vi "Actor Core.vi"(8 "error in":errorcluster, 11 "Nested in":refnum<class "MQTT_Client_Actor.lvclass">) -> (0 "error out":errorcluster, 3 "Actor out":refnum<class "Actor.lvclass">)   [LabVIEW 2018, in "MQTT_Client_Actor.lvlib" / "MQTT_Client_Actor.lvclass"]
doc: "(<B>Filename</B>: Actor Framework.lvlib:Actor.lvclass:Actor Core.vi)\n\nReceives messages to the actor, reacts to them, and initiates any error handling that may shut the actor down.\n\nDescendant classes may override this VI to append parallel tasks for the actor to complete while it handles messages. Overrides use the Call Parent Method node."
uses:
  MQTT_Client_Actor.lvclass
  D:/Program Files (x86)/National Instruments/LabVIEW 2018/vi.lib/ActorFramework/Actor/Actor.lvclass
  <vilib>/ActorFramework/Actor/Actor.lvclass
  CreateClient.ctl
  <vilib>/LabVIEW Open Source Project/MQTT Control Packets/Control Packets/ControlPacket/QualityOfService -- enum.ctl
  <vilib>/LabVIEW Open Source Project/MQTT Client/Client class/Client.lvclass
  D:/Program Files (x86)/National Instruments/LabVIEW 2018/vi.lib/LabVIEW Open Source Project/MQTT Connection/MQTT_Base/Base Class/MQTT_Base.lvclass
  MQTT_Client_Actor.lvclass/MQTT_Client_Actor.ctl
  <vilib>/ActorFramework/Actor/Actor.lvclass/Actor.ctl
  <vilib>/ActorFramework/Message Enqueuer/Message Enqueuer.lvclass/Message Enqueuer.ctl
  <vilib>/LabVIEW Open Source Project/MQTT Client/Client class/Client.lvclass/Client.ctl
  <vilib>/LabVIEW Open Source Project/MQTT Connection/MQTT_Base/Base Class/MQTT_Base.lvclass/MQTT_Base.ctl
  <vilib>/LabVIEW Open Source Project/MQTT Control Packets/Control Packets/ControlPacket/ControlPacket.lvclass/ControlPacket.ctl
  <vilib>/LabVIEW Open Source Project/MQTT Control Packets/Control Packets/CONNECT/ConnectFlags -- cluster.ctl
  SubscribeClient.ctl
  PublishClient.ctl
  <vilib>/ActorFramework/Message Enqueuer/Init from Existing Queue.vi
  <vilib>/ActorFramework/Message Enqueuer/Enqueue.vi
  <vilib>/ActorFramework/Stop Msg/Stop Msg.lvclass
  D:/Program Files (x86)/National Instruments/LabVIEW 2018/vi.lib/ActorFramework/Message/Message.lvclass
  <vilib>/LabVIEW Open Source Project/MQTT Control Packets/Control Packets/PUBLISH/PUBLISH.lvclass
  D:/Program Files (x86)/National Instruments/LabVIEW 2018/vi.lib/LabVIEW Open Source Project/MQTT Control Packets/Control Packets/ControlPacket/ControlPacket.lvclass
  <vilib>/LabVIEW Open Source Project/Connection/Connection.TCP/Connection.TCP.lvclass
  D:/Program Files (x86)/National Instruments/LabVIEW 2018/vi.lib/LabVIEW Open Source Project/Connection/Connection/Connection.lvclass
  <vilib>/ActorFramework/Message Priority Queue/Priority Enqueue.vi
  <vilib>/ActorFramework/Message Enqueuer/Message Enqueuer.lvclass
  <vilib>/LabVIEW Open Source Project/MQTT Connection/MQTT_Base/Base Class/MQTT_Base.lvclass
  <vilib>/LabVIEW Open Source Project/MQTT Control Packets/Control Packets/ControlPacket/ControlPacket.lvclass
  MQTT_Client_Actor Messages/1_CreateClient Msg/1_CreateClient Msg.lvclass
  <vilib>/LabVIEW Open Source Project/MQTT Control Packets/Control Packets/CONNECT/CONNECT.lvclass
  MQTT_Client_Actor Messages/2_Subscribe Msg/2_Subscribe Msg.lvclass
  MQTT_Client_Actor Messages/3_UpdateSubscribeList Msg/3_UpdateSubscribeList Msg.lvclass
  MQTT_Client_Actor Messages/4_Publish Msg/4_Publish Msg.lvclass
panel:
  in  "RETAIN":bool
  out "SubscribeLists":i32(listbox)
  in  "Topic Name":string="Topic"
  in  "QoS":T1=enum."1 (At Least Once)"
  in  "Create":T2={"address"="localhost", "port"=1883, "UserName"="", "Pwd"=""}
  out "ServerStatus":bool
  in  "CreateClient":bool
  in  "UnSubscribe":bool
  out "ReceivedData":i32(listbox)
  in  "Subscribe":bool
  in  "Publish":bool
  out "Published":bool
  in  "Data":string="12345"
  in  "DisConnect":bool
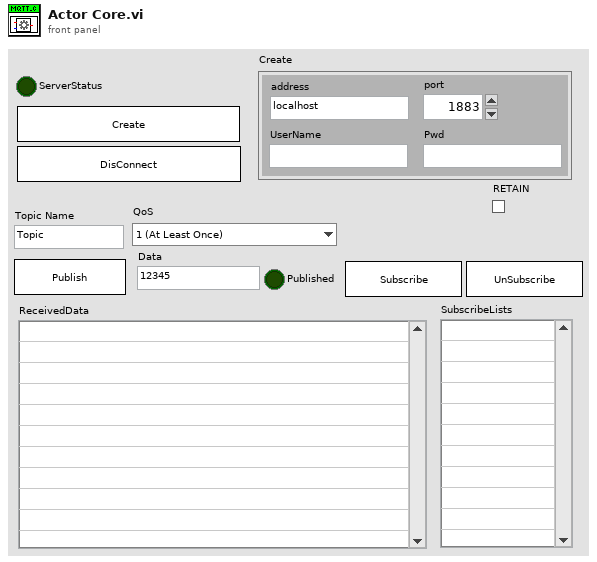
[diagram p1: front panel]
types:
  T1 = typedef "MQTT_Control_Packets.lvlib/ControlPacket.lvclass/QualityOfService -- enum.ctl" = enum16{"0 (At Most Once)", "1 (At Least Once)", "2 (Exactly Once)"}
  T2 = typedef "MQTT_Client_Actor.lvlib/MQTT_Client_Actor.lvclass/CreateClient.ctl" = cluster{"address":string, "port":u16, "UserName":string, "Pwd":string}
  T3 = typedef "MQTT Client.lvlib/Client.lvclass/Public Events -- cluster.ctl" = cluster{"Connection Status":refnum<user-event>, "Connected":refnum<user-event>, "Application Message":refnum<user-event>}
  T4 = cluster{"Stop":refnum<user-event>, "Create":refnum<user-event>, "Subscribe":refnum<user-event>, "Init":refnum<user-event>, "Publish":refnum<user-event>}
  T5 = typedef "MQTT Base.lvlib/MQTT_Base.lvclass/Public Events -- cluster.ctl" = cluster{"Stop Event":refnum<user-event>, "Error Event":refnum<user-event>, "Inbound Message":refnum<user-event>}
  T6 = typedef "MQTT_Control_Packets.lvlib/CONNECT.lvclass/ConnectFlags -- cluster.ctl" = cluster{"Reserved":bool, "Clean Session":bool, "Will Flag":bool, "Will QoS 1":bool, "Will QoS 2":bool, "Will Retain":bool, "Password Flag":bool, "User Name Flag":bool}
  T7 = cluster{"Will Topic":string, "Will Message":string, "Username":string, "Password":string}
  T8 = typedef "MQTT_Client_Actor.lvlib/MQTT_Client_Actor.lvclass/SubscribeClient.ctl" = cluster{"Topic Name":string, "QoS":T1, "T:Subscribe":bool}
  T9 = typedef "MQTT_Client_Actor.lvlib/MQTT_Client_Actor.lvclass/PublishClient.ctl" = cluster{"Topic Name":string, "QoS":T1, "RETAIN":bool, "Topic Data":string}
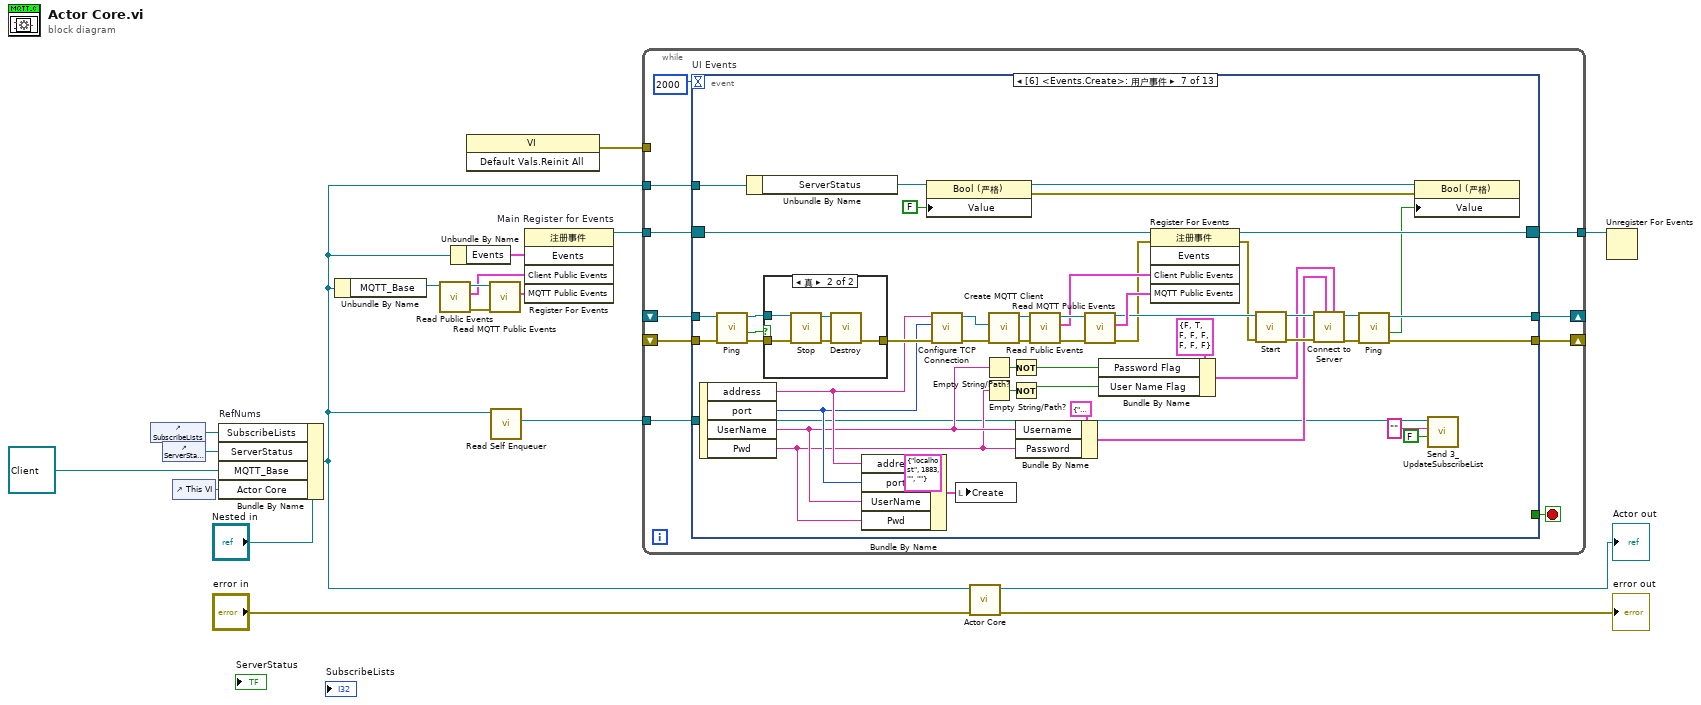
[diagram p0: block diagram]
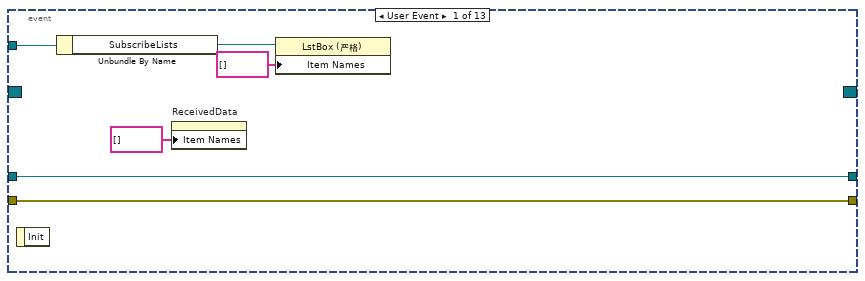
[diagram p2: hidden frame]
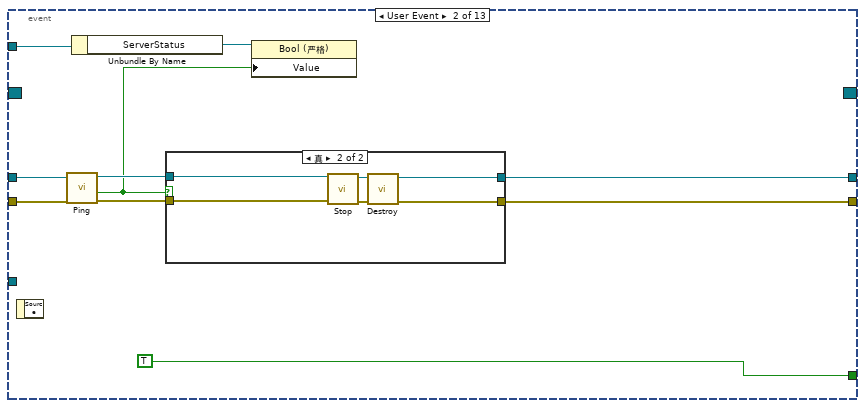
[diagram p3: hidden frame]
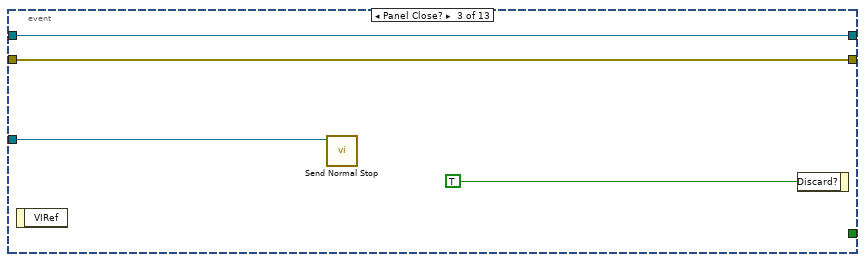
[diagram p5: hidden frame]
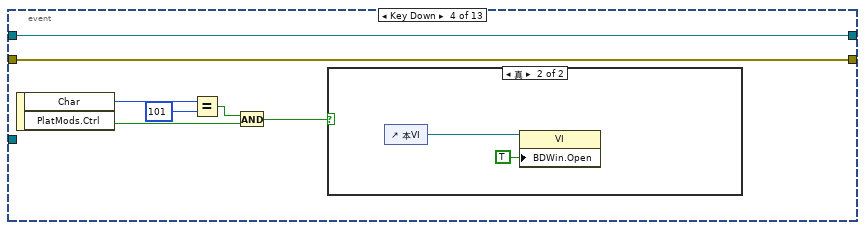
[diagram p6: hidden frame]
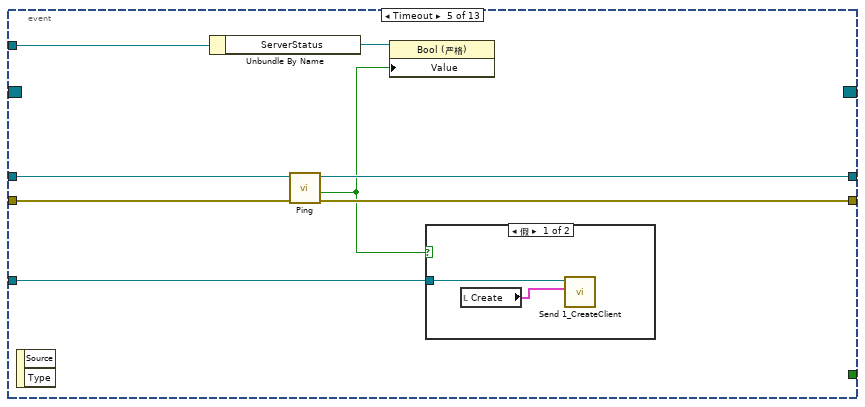
[diagram p8: hidden frame]
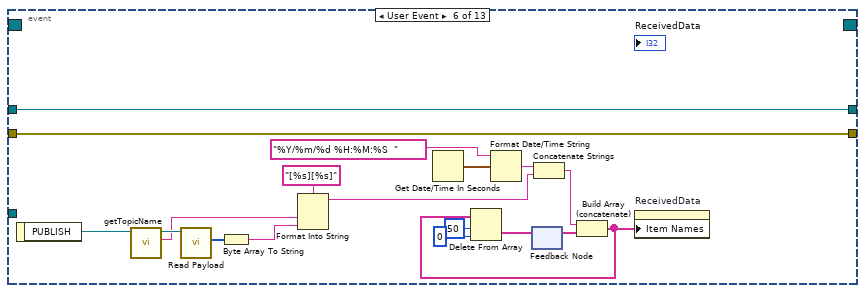
[diagram p10: hidden frame]
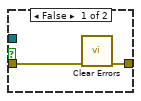
[diagram p11: hidden frame]
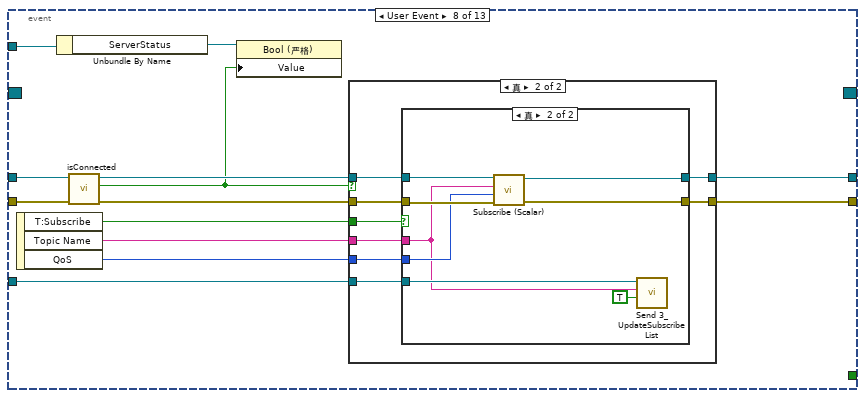
[diagram p12: hidden frame]
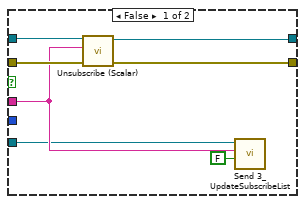
[diagram p14: hidden frame]
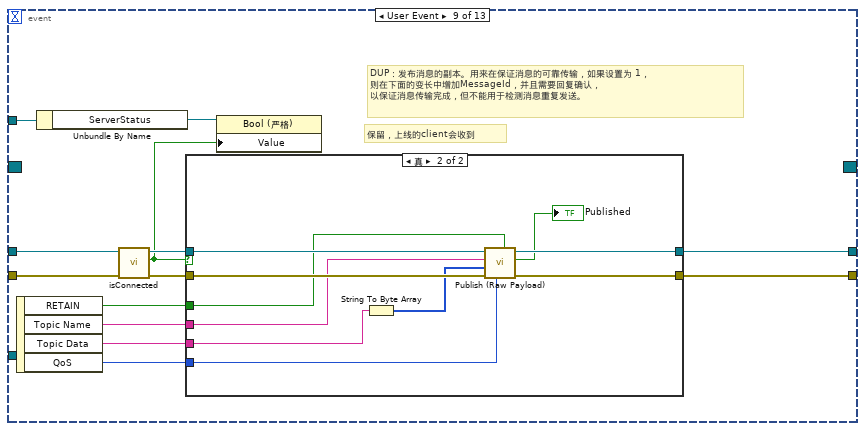
[diagram p15: hidden frame]
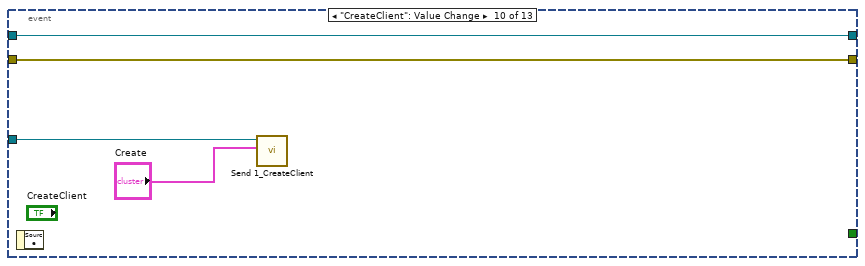
[diagram p17: hidden frame]
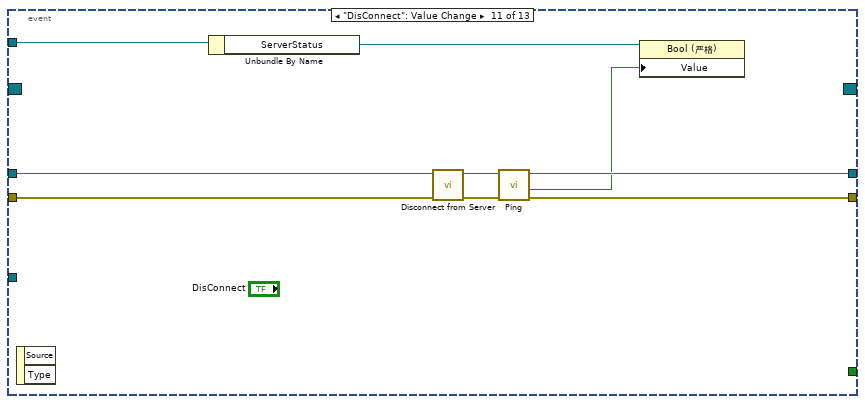
[diagram p18: hidden frame]
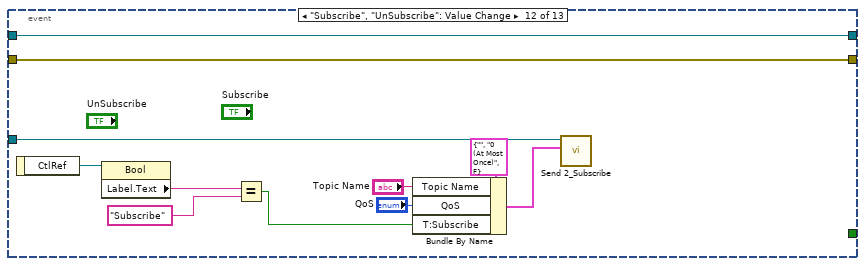
[diagram p19: hidden frame]
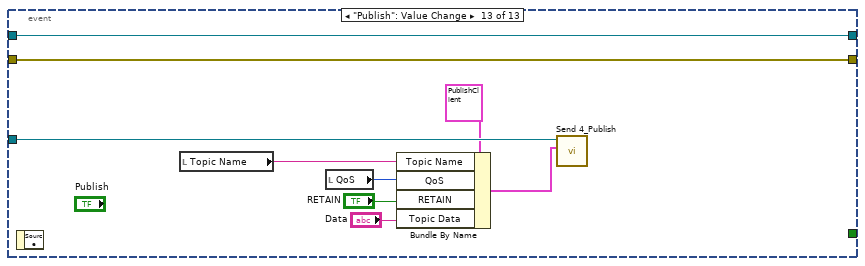
[diagram p20: hidden frame]
diagram:
  n1 = control-ref of="SubscribeLists"() -> (w2:refnum<vi>)
  n2 = control-ref of="ServerStatus"() -> (w4:refnum<vi>)
  n3 = control-ref of="This VI"() -> (w12:refnum<vi>)
  n4 = Bundle By Name "RefNums"(cluster="Nested in", "SubscribeLists"=w2, "ServerStatus"=w4, "MQTT_Base"=refnum<class "Client.lvclass"> refnum, "Actor Core"=w12) -> (w3:refnum<class "MQTT_Client_Actor.lvclass">)
  n5 = Unbundle By Name(w3) -> ("MQTT_Base"=w7:refnum<class "Client.lvclass">)
  n6 = call <vilib>:"Read Public Events.vi"("Client in"=w7) -> ("error out"=w8:errorcluster, "Client Public Events"=w6:T3, "Client out"=w9:refnum<class "Client.lvclass">)  [unwired: 8 in]
  n7 = Unbundle By Name(w3) -> ("Events"=w16:T4)
  n8 = invoke class="VI" method="Default Vals.Reinit All"() -> (error out=w1:errorcluster)  [unwired: 3 in, 2 out]
  n9 = call <vilib>:"Read MQTT Public Events.vi"("error in (no error)"=w8, "MQTT_Base in"=w9) -> ("MQTT Public Events"=w5:T5)  [unwired: 7 in, 2 out]
  n10 = call <vilib>:"Read Self Enqueuer.vi"("Actor"=w3) -> ("Self Enqueuer"=w14:refnum<class "Message Enqueuer.lvclass">)  [unwired: 10 in]
  n11 = register-events "Main Register for Events"(w16, w6, w5) -> (reference out=w17:refnum<event-registration>)  [unwired: 2 in, 1 out]
  n12 = while {
    tunnel: w17 -> [w29]
    tunnel: [w27] -> w15
    tunnel: w14 -> [w26]
    shift-right: [w25] -> _
    shift-left: _ -> [w21]
    shift-right: [w24] -> _
    shift-left: _ -> [w22]
    tunnel: w3 -> [w20]
    tunnel: w1 -> [_]
    stop <- w28 stop-if-true
    n13 = event "UI Events" shown="[6] <Events.Create>: 用户事件" {
      selector: w29 -> [_ _ _ _ _ _ w137 _ _ _ _ _ _]
      dyn-events: [_ _ _ _ _ _ w134 _ _ _ _ _ _] -> w27
      timeout: 2000 -> [_ _ _ _ _ _ _ _ _ _ _ _ _]
      tunnel: [_ TRUE _ _ _ _ _ _ _ _ _ _ _] -> w28
      tunnel: w26 -> [_ _ w56 _ w68 _ w95 w150 _ w213 _ w234 w243]
      tunnel: [w35 w40 w54 w64 w72 w91 w110 w157 w195 w216 w220 w236 w245] -> w25
      tunnel: [w34 w39 w55 w63 w71 w90 w125 w158 w196 w215 w221 w235 w244] -> w24
      tunnel: w22 -> [w34 w44 w55 w63 w74 w90 w123 w160 w198 w215 w225 w235 w244]
      tunnel: w21 -> [w35 w43 w54 w64 w73 w91 w122 w159 w197 w216 w224 w236 w245]
      tunnel: w20 -> [w32 w37 _ _ w69 _ w116 w155 w193 _ w218 _ _]
      event User Event {
        n14 = event-data() -> ()  [unwired: 1 in, 1 out]
        n15 = Unbundle By Name(w32) -> ("SubscribeLists"=w31:refnum<vi>)
        n16 = property on="ReceivedData" class="LstBox (严格)"("Item Names"=string[] [] ("项名")) -> ()  [unwired: 2 in, 2 out]
        n17 = property class="LstBox (严格)"(reference=w31, "Item Names"=string[] [] ("项名")) -> ()  [unwired: 1 in, 2 out]
      }
      event User Event {
        n18 = event-data() -> ()  [unwired: 1 in, 1 out]
        n19 = call <vilib>:"Ping.vi"("error in (no error)"=w43, "Client in"=w44) -> ("error out"=w41:errorcluster, "Server responded"=w36:bool, "Client out"=w42:refnum<class "Client.lvclass">)  [unwired: 6 in, 1 out]
        n20 = Unbundle By Name(w37) -> ("ServerStatus"=w38:refnum<vi>)
        n21 = case shown="真" w36 {
          tunnel: w42 -> [w47 w51]
          tunnel: w41 -> [w46 w50]
          tunnel: [w46 w49] -> w40
          tunnel: [w47 w48] -> w39
          frame False {
          }
          frame True {
            n22 = call <vilib>:"Stop.vi"("error in (no error)"=w50, "MQTT_Base in"=w51) -> ("error out"=w52:errorcluster, "MQTT_Base out"=w53:refnum<class "Client.lvclass">)  [unwired: 7 in, 1 out]
            n23 = call <vilib>:"Destroy.vi"("error in (no error)"=w52, "MQTT_Base in"=w53) -> ("error out"=w49:errorcluster, "MQTT_Base out"=w48:refnum<class "Client.lvclass">)  [unwired: 8 in]
          }
        }
        n24 = property class="Bool (严格)"(reference=w38, "Value"=w36) -> ()  [unwired: 1 in, 2 out]
      }
      event Panel Close? {
        n25 = event-data() -> ()  [unwired: 1 in, 1 out]
        n26 = call <vilib>:"Send Normal Stop.vi"("Message Enqueuer"=w56) -> ()  [unwired: 10 in, 1 out]
        n27 = event-data("Discard?"=TRUE) -> ()  [unwired: 1 in, 1 out]
      }
      event Key Down {
        n28 = event-data() -> ("Char"=w59:i16, "PlatMods.Ctrl"=w58:bool)  [unwired: 1 in]
        n29 = Equal?(x=w59, y=i16 101) -> (x = y?=w61:bool)
        n30 = And(x=w61, y=w58) -> (x .and. y?=w60:bool)
        n31 = case shown="真" w60 {
          frame False {
          }
          frame True {
            n32 = control-ref of="本VI"() -> (w66:refnum<vi>)
            n33 = property class="VI"(reference=w66, "BDWin.Open"=TRUE ("程序框图窗口:打开")) -> ()  [unwired: 1 in, 2 out]
          }
        }
      }
      event Timeout {
        n34 = event-data() -> ()  [unwired: 1 in, 2 out]
        n35 = Unbundle By Name(w69) -> ("ServerStatus"=w70:refnum<vi>)
        n36 = call <vilib>:"Ping.vi"("error in (no error)"=w73, "Client in"=w74) -> ("error out"=w72:errorcluster, "Server responded"=w67:bool, "Client out"=w71:refnum<class "Client.lvclass">)  [unwired: 6 in, 1 out]
        n37 = property class="Bool (严格)"(reference=w70, "Value"=w67) -> ()  [unwired: 1 in, 2 out]
        n38 = case shown="假" w67 {
          tunnel: w68 -> [w76 _]
          frame False {
            n39 = local read "Create"() -> (w75:T2)
            n40 = call "Send 1_CreateClient.vi"("Create"=w75, "Message Enqueuer in"=w76) -> ()  [unwired: 8 in, 2 out]
          }
          frame True {
          }
        }
      }
      event User Event {
        n41 = event-data() -> ("PUBLISH"=w92:refnum<class "PUBLISH.lvclass">)  [unwired: 1 in]
        n42 = call <vilib>:"getTopicName.vi"("PUBLISH in"=w92) -> ("Topic"=w80:string, "PUBLISH out"=w93:refnum<class "PUBLISH.lvclass">)  [unwired: 8 in, 1 out]
        n43 = call <vilib>:"Read Payload.vi"("ControlPacket in"=w93) -> ("Payload"=w94:u8[])  [unwired: 9 in, 1 out]
        n44 = Byte Array To String(unsigned byte array=w94) -> (string=w79:string)
        n45 = Format Into String(format string="[%s][%s]" ("格式字符串"), w80, w79) -> (resulting string=w77:string)  [unwired: 2 in, 1 out]
        n46 = Get Date/Time In Seconds() -> (seconds since 1Jan1904=w89:timestamp)
        n47 = Format Date/Time String(time format string (%c)="%Y/%m/%d %H:%M:%S  " ("时间格式字符串(%c)"), seconds (now)=w89) -> (date/time string=w88:string)  [unwired: 1 in]
        n48 = feedback #1() -> (w85:string[])  [unwired: 1 in]
        n49 = Concatenate Strings(w88, w77) -> (w86:string)
        n50 = Build Array (concatenate)(w86, w85) -> (w81:string[])
        n51 = Delete From Array(array=w81, length=50 ("长度"), index=0 ("索引")) -> (deleted portion=w82:string[])  [unwired: 1 out]
        n52 = feedback-in #1(w82) -> ()
        n53 = property on="ReceivedData" class="LstBox (严格)"("Item Names"=w81) -> ()  [unwired: 2 in, 2 out]
      }
      event User Event {
        n54 = event-data() -> ("address"=w101:string, "port"=w100:u16, "UserName"=w99:string, "Pwd"=w98:string)  [unwired: 1 in]
        n55 = call <vilib>:"Ping.vi"("error in (no error)"=w122, "Client in"=w123) -> ("error out"=w119:errorcluster, "Server responded"=w121:bool, "Client out"=w120:refnum<class "Client.lvclass">)  [unwired: 6 in, 1 out]
        n56 = Unbundle By Name(w116) -> ("ServerStatus"=w114:refnum<vi>)
        n57 = case shown="真" w121 {
          tunnel: [w143 w147] -> w129
          tunnel: w120 -> [_ w146]
          tunnel: w119 -> [w144 w145]
          frame False {
            n58 = call <vilib>:"Clear Errors.vi"("error in (no error)"=w144) -> ("error out"=w143:errorcluster)  [unwired: 5 in, 1 out]
          }
          frame True {
            n59 = call <vilib>:"Stop.vi"("error in (no error)"=w145, "MQTT_Base in"=w146) -> ("error out"=w148:errorcluster, "MQTT_Base out"=w149:refnum<class "Client.lvclass">)  [unwired: 7 in, 1 out]
            n60 = call <vilib>:"Destroy.vi"("error in (no error)"=w148, "MQTT_Base in"=w149) -> ("error out"=w147:errorcluster)  [unwired: 8 in, 1 out]
          }
        }
        n61 = Bundle By Name(cluster=T2 {"address"="localhost", "port"=1883, "UserName"="", "Pwd"=""} ("Create"), "address"=w101, "port"=w100, "UserName"=w99, "Pwd"=w98) -> (w102:T2)
        n62 = property class="Bool (严格)"(reference=w114, "Value"=FALSE ("值")) -> (reference out=w113:refnum<vi>, error out=w112:errorcluster)  [unwired: 1 in]
        n63 = call <vilib>:"Configure TCP Connection.vi"("error in (no error)"=w129, "remote port (80)"=w100, "address (localhost)"=w101) -> ("error out"=w133:errorcluster, "Connection.TCP"=w138:refnum<class "Connection.TCP.lvclass">)  [unwired: 7 in]
        n64 = local write "Create"(w102) -> ()
        n65 = Empty String/Path?(string/path=w99) -> (empty?=w107:bool)
        n66 = Empty String/Path?(string/path=w98) -> (empty?=w106:bool)
        n67 = call <vilib>:"Create MQTT Client.vi"("error in (no error)"=w133, "Connection Configuration"=w138) -> ("error out"=w140:errorcluster, "Client out"=w142:refnum<class "Client.lvclass">)  [unwired: 8 in]
        n68 = Not(x=w107) -> (.not. x?=w105:bool)
        n69 = Not(x=w106) -> (.not. x?=w104:bool)
        n70 = Bundle By Name(cluster=T7 {"Will Topic"="", "Will Message"="", "Username"="", "Password"=""} ("Payload"), "Username"=w99, "Password"=w98) -> (w117:T7)
        n71 = call <vilib>:"Read Public Events.vi"("error in (no error)"=w140, "Client in"=w142) -> ("error out"=w139:errorcluster, "Client Public Events"=w136:T3, "Client out"=w141:refnum<class "Client.lvclass">)  [unwired: 7 in]
        n72 = call <vilib>:"Read MQTT Public Events.vi"("error in (no error)"=w139, "MQTT_Base in"=w141) -> ("error out"=w130:errorcluster, "MQTT Public Events"=w135:T5, "MQTT_Base out"=w132:refnum<class "Client.lvclass">)  [unwired: 7 in]
        n73 = Bundle By Name(cluster=T6 {"Reserved"=FALSE, "Clean Session"=TRUE, "Will Flag"=FALSE, "Will QoS 1"=FALSE, "Will QoS 2"=FALSE, "Will Retain"=FALSE, "Password Flag"=FALSE, "User Name Flag"=FALSE} ("Connect Flags"), "Password Flag"=w105, "User Name Flag"=w104) -> (w108:T6)
        n74 = register-events ("Main Register for Events")(reference=w137, error in=w130, w136, w135) -> (reference out=w134:refnum<event-registration>, error out=w131:errorcluster)  [unwired: 1 in]
        n75 = call <vilib>:"Start.vi"("error in (no error)"=w131, "MQTT_Base in"=w132) -> ("error out"=w127:errorcluster, "MQTT_Base out"=w128:refnum<class "Client.lvclass">)  [unwired: 7 in, 1 out]
        n76 = call <vilib>:"Connect to Server.vi"("Connect Flags"=w108, "Payload"=w117, "error in (no error)"=w127, "Client in"=w128) -> ("error out"=w124:errorcluster, "Client out"=w126:refnum<class "Client.lvclass">)  [unwired: 4 in, 2 out]
        n77 = call <vilib>:"Ping.vi"("error in (no error)"=w124, "Client in"=w126) -> ("error out"=w110:errorcluster, "Server responded"=w115:bool, "Client out"=w125:refnum<class "Client.lvclass">)  [unwired: 6 in, 1 out]
        n78 = property class="Bool (严格)"(reference=w113, error in=w112, "Value"=w115) -> ()  [unwired: 2 out]
        n79 = call "Send 3_UpdateSubscribeList.vi"("T:Add"=FALSE, "Topic"="", "Message Enqueuer in"=w95) -> ()  [unwired: 7 in, 2 out]
      }
      event User Event {
        n80 = event-data() -> ("T:Subscribe"=w153:bool, "Topic Name"=w152:string, "QoS"=w151:T1)  [unwired: 1 in]
        n81 = Unbundle By Name(w155) -> ("ServerStatus"=w156:refnum<vi>)
        n82 = call <vilib>:"isConnected.vi"("error in (no error)"=w159, "Client in"=w160) -> ("error out"=w161:errorcluster, "connected"=w154:bool, "Client out"=w162:refnum<class "Client.lvclass">)  [unwired: 7 in]
        n83 = property class="Bool (严格)"(reference=w156, "Value"=w154) -> ()  [unwired: 1 in, 2 out]
        n84 = case shown="真" w154 {
          tunnel: w162 -> [w164 w172]
          tunnel: w161 -> [w163 w171]
          tunnel: [w164 w170] -> w158
          tunnel: [w163 w169] -> w157
          tunnel: w153 -> [_ w168]
          tunnel: w152 -> [_ w167]
          tunnel: w151 -> [_ w166]
          tunnel: w150 -> [_ w165]
          frame False {
          }
          frame True {
            n85 = case shown="真" w168 {
              tunnel: [w177 w186] -> w170
              tunnel: [w176 w185] -> w169
              tunnel: w172 -> [w179 w187]
              tunnel: w171 -> [w178 w184]
              tunnel: w167 -> [w174 w180]
              tunnel: w166 -> [_ w183]
              tunnel: w165 -> [w173 w182]
              frame False {
                n86 = call <vilib>:"Unsubscribe (Scalar).vi"("error in (no error)"=w178, "Topic Filter"=w174, "Client in"=w179) -> ("error out"=w176:errorcluster, "Client out"=w177:refnum<class "Client.lvclass">)  [unwired: 6 in, 1 out]
                n87 = call "Send 3_UpdateSubscribeList.vi"("T:Add"=FALSE, "Topic"=w174, "Message Enqueuer in"=w173) -> ()  [unwired: 7 in, 2 out]
              }
              frame True {
                n88 = call <vilib>:"Subscribe (Scalar).vi"("error in (no error)"=w184, "QoS"=w183, "Topic Filter"=w180, "Client in"=w187) -> ("error out"=w185:errorcluster, "Client out"=w186:refnum<class "Client.lvclass">)  [unwired: 5 in, 1 out]
                n89 = call "Send 3_UpdateSubscribeList.vi"("T:Add"=TRUE, "Topic"=w180, "Message Enqueuer in"=w182) -> ()  [unwired: 7 in, 2 out]
              }
            }
          }
        }
      }
      event User Event {
        # "保留，上线的client会收到"
        # "DUP：发布消息的副本。用来在保证消息的可靠传输，如果设置为 1，\n则在下面的变长中增加MessageId，并且需要回复确认，\n以保证消息传输完成，但不能用于检测消息重复发送。"
        n90 = event-data() -> ("RETAIN"=w191:bool, "Topic Name"=w190:string, "Topic Data"=w189:string, "QoS"=w188:T1)  [unwired: 1 in]
        n91 = Unbundle By Name(w193) -> ("ServerStatus"=w194:refnum<vi>)
        n92 = call <vilib>:"isConnected.vi"("error in (no error)"=w197, "Client in"=w198) -> ("error out"=w200:errorcluster, "connected"=w192:bool, "Client out"=w199:refnum<class "Client.lvclass">)  [unwired: 7 in]
        n93 = case shown="真" w192 {
          tunnel: [w202 w211] -> w196
          tunnel: [w201 w210] -> w195
          tunnel: w199 -> [w202 w212]
          tunnel: w200 -> [w201 w209]
          tunnel: w191 -> [_ w206]
          tunnel: w190 -> [_ w205]
          tunnel: w189 -> [_ w204]
          tunnel: w188 -> [_ w203]
          frame False {
          }
          frame True {
            n94 = String To Byte Array(string=w204) -> (unsigned byte array=w208:u8[])
            n95 = call <vilib>:"Publish (Raw Payload).vi"("RETAIN"=w206, "QoS"=w203, "error in (no error)"=w209, "Binary Payload"=w208, "Topic Name"=w205, "Client in"=w212) -> ("error out"=w210:errorcluster, "Published"=→"Published":bool, "Client out"=w211:refnum<class "Client.lvclass">)  [unwired: 3 in]
          }
        }
        n96 = property class="Bool (严格)"(reference=w194, "Value"=w192) -> ()  [unwired: 1 in, 2 out]
      }
      event "CreateClient": Value Change {
        n97 = event-data() -> ()  [unwired: 1 in, 1 out]
        n98 = call "Send 1_CreateClient.vi"("Create"="Create", "Message Enqueuer in"=w213) -> ()  [unwired: 8 in, 2 out]
      }
      event "DisConnect": Value Change {
        n99 = event-data() -> ()  [unwired: 1 in, 2 out]
        n100 = Unbundle By Name(w218) -> ("ServerStatus"=w219:refnum<vi>)
        n101 = call <vilib>:"Disconnect from Server.vi"("error in (no error)"=w224, "Client in"=w225) -> ("error out"=w222:errorcluster, "Client out"=w223:refnum<class "Client.lvclass">)  [unwired: 7 in, 1 out]
        n102 = call <vilib>:"Ping.vi"("error in (no error)"=w222, "Client in"=w223) -> ("error out"=w220:errorcluster, "Server responded"=w217:bool, "Client out"=w221:refnum<class "Client.lvclass">)  [unwired: 6 in, 1 out]
        n103 = property class="Bool (严格)"(reference=w219, "Value"=w217) -> ()  [unwired: 1 in, 2 out]
      }
      event "Subscribe", "UnSubscribe": Value Change {
        n104 = event-data() -> ("CtlRef"=w233:refnum<vi>)  [unwired: 1 in]
        n105 = property class="Bool"(reference=w233) -> ("Label.Text"=w232:string)  [unwired: 1 in, 2 out]
        n106 = Equal?(x=w232, y="Subscribe") -> (x = y?=w226:bool)
        n107 = Bundle By Name(cluster=T8 {"Topic Name"="", "QoS"=enum."0 (At Most Once)", "T:Subscribe"=FALSE} ("Subscribe"), "Topic Name"="Topic Name", "QoS"="QoS", "T:Subscribe"=w226) -> (w229:T8)
        n108 = call "Send 2_Subscribe.vi"("Subscribe"=w229, "Message Enqueuer in"=w234) -> ()  [unwired: 8 in, 2 out]
      }
      event "Publish": Value Change {
        n109 = event-data() -> ()  [unwired: 1 in, 1 out]
        n110 = local read "Topic Name"() -> (w240:string)
        n111 = local read "QoS"() -> (w239:T1)
        n112 = Bundle By Name(cluster=T9 {"Topic Name"="TopicA", "QoS"=enum."1 (At Least Once)", "RETAIN"=FALSE, "Topic Data"=""} ("Subscribe"), "Topic Name"=w240, "QoS"=w239, "RETAIN"="RETAIN", "Topic Data"="Data") -> (w241:T9)
        n113 = call "Send 4_Publish.vi"("Subscribe"=w241, "Message Enqueuer in"=w243) -> ()  [unwired: 8 in, 2 out]
      }
    }
  }
  n114 = call-parent "Actor Core.vi"("error in"="error in", "Actor in"=w3) -> ("error out"=→"error out":errorcluster, "Actor out"=→"Actor out":refnum<class "Actor.lvclass">)  [unwired: 8 in]
  n115 = Unregister For Events(event registration refnum=w15) -> ()  [unwired: 1 in, 1 out]
